vi "Create Message.vi"(8 "error in":errorcluster, 9 "Client ID":string, 10 "Topic.lvclass":refnum<class "Topic.lvclass">, 11 "Message in":refnum<class "Message.lvclass">) -> (0 "error out":errorcluster, 3 "Message out":refnum<class "Message.lvclass">)   [LabVIEW 2014, in "Message.lvclass"]
uses:
  Message.lvclass
  Topic_class/Topic.lvclass
  Message.lvclass/Message.ctl
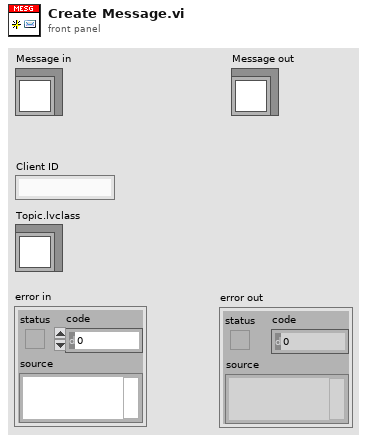
[diagram p1: front panel]
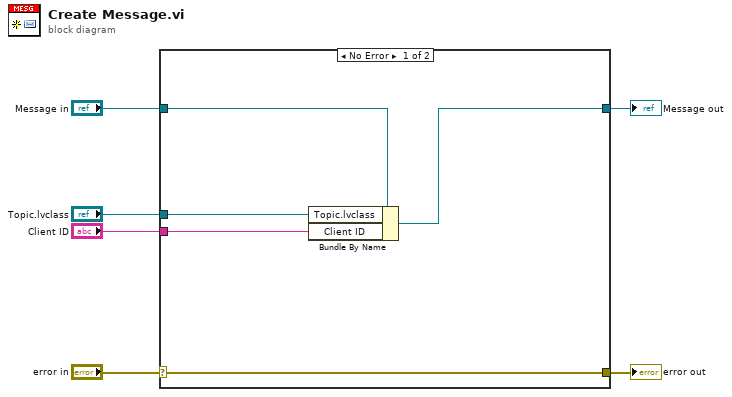
[diagram p0: block diagram]
diagram:
  n1 = case shown="No Error" "error in" {
    selector: "error in" -> [w11 w13]
    tunnel: [w11 w13] -> w5
    tunnel: [w9 w12] -> w3
    tunnel: "Message in" -> [w10 w12]
    tunnel: "Topic.lvclass" -> [w8 _]
    tunnel: "Client ID" -> [w7 _]
    frame No Error {
      n2 = Bundle By Name(cluster=w10, "Topic.lvclass"=w8, "Client ID"=w7) -> (w9:refnum<class "Message.lvclass">)
    }
    frame Error {
    }
  }
  "error out" <- w5
  "Message out" <- w3
